vi "device on off list mouse down.vi"(6 "Button":u16, 7 "Coords":T1, 9 "Array 2":i32[](array[numeric]), 10 "CtlRef":refnum<vi>, 11 "Array in":refnum<vi>) -> (2 "Array":bool[](array[boolean]), 3 "ItemSyms":i32[](array[numeric]))   [LabVIEW 2018]
uses:
  <vilib>/Utility/miscctls.llb/LVPoint32TypeDef.ctl
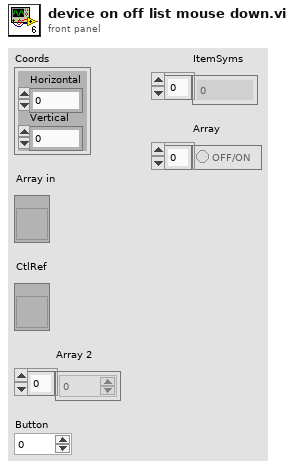
[diagram p1: front panel]
types:
  T1 = typedef "LVPoint32TypeDef.ctl" = cluster{"Horizontal":i32, "Vertical":i32}
  T2 = enum8{"Enabled", "Disabled", "Disabled and Grayed Out"}
  T3 = typedef "mysql_authentication.ctl" = cluster{"User":string, "Password":string, "Database":string}
  T4 = cluster{"Port":u16, "IP Address":string, "Authentication":T3}
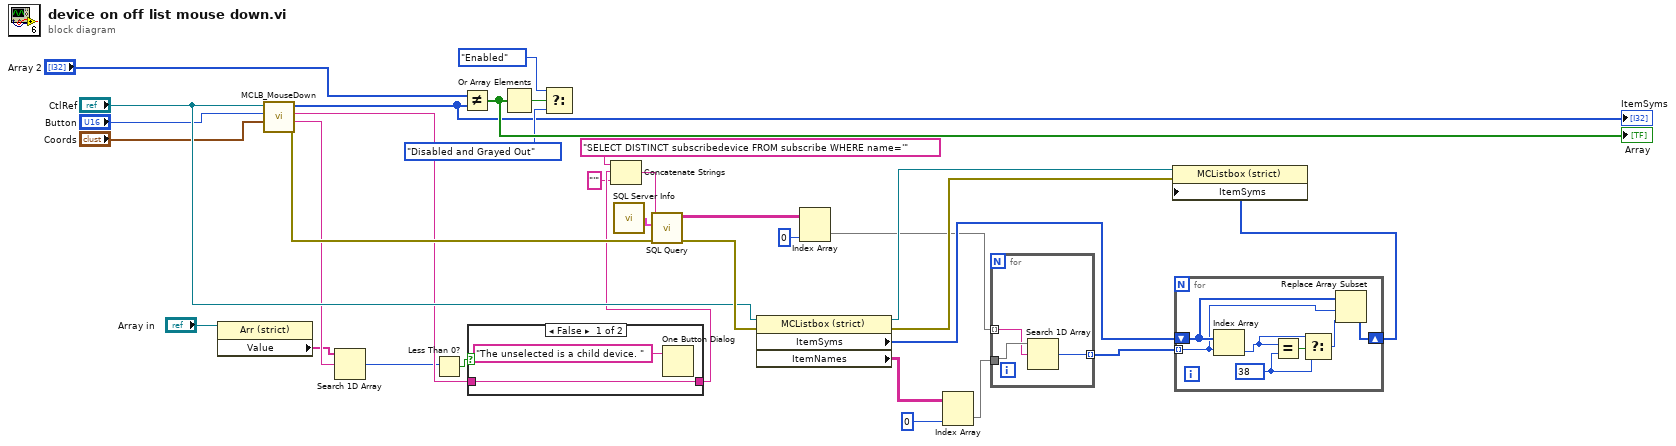
[diagram p0: block diagram]
diagram:
  n1 = property class="Arr (strict)"(reference="Array in") -> ("Value"=w10:string[])  [unwired: 1 in, 2 out]
  n2 = call "MCLB_MouseDown.vi"("Coords"="Coords", "Button"="Button", "MCListbox Refnum"="CtlRef") -> ("error out"=w31:errorcluster, "Unselected Item"=w11:string, "Selected Item"=w13:string, "ItemSyms"=w4:i32[])  [unwired: 5 in]
  "ItemSyms" <- w4
  n3 = Search 1D Array(1D array=w10, element=w11) -> (index of element=w9:i32)  [unwired: 1 in]
  n4 = Less Than 0?(x=w9) -> (x < 0?=w12:bool)
  n5 = Not Equal?(x="Array 2", y=w4) -> (x != y?=w8:bool[])
  "Array" <- w8
  n6 = case shown="False" w12 {
    tunnel: w13 -> [w35 w36]
    tunnel: [w35 w36] -> w20
    frame False {
      n7 = One Button Dialog(message="The unselected is a child device. ") -> ()  [unwired: 1 in, 1 out]
    }
    frame True {
    }
  }
  n8 = Or Array Elements(Boolean array=w8) -> (logical OR=w33:bool)
  n9 = Select(t=T2."Enabled" ("Disabled"), s=w33, f=T2."Disabled and Grayed Out" ("Disabled")) -> ()  [unwired: 1 out]
  n10 = Concatenate Strings("SELECT DISTINCT subscribedevice FROM subscribe WHERE name='" ("Query"), w20, "'" ("string")) -> (w16:string)
  n11 = call "SQL Server Info.vi"() -> ("SQL Server Info"=w19:T4)
  n12 = call "SQL Query.vi"("error in (no error)"=w31, "SQL Server Info"=w19, "Query"=w16) -> ("error out"=w32:errorcluster, "data"=w15:string[][])  [unwired: 7 in]
  n13 = property class="MCListbox (strict)"(reference="CtlRef", error in=w32) -> (reference out=w28:refnum<vi>, error out=w29:errorcluster, "ItemSyms"=w26:i32[], "ItemNames"=w24:string[][])
  n14 = Index Array(array=w15, index (col)=0 ("disabled index (col)")) -> (element=w25:string[])  [unwired: 1 in]
  n15 = Index Array(array=w24, index (col)=0 ("disabled index (col)")) -> (element=w22:string[])  [unwired: 1 in]
  n16 = for {
    tunnel: w25 -> [w38] mode=indexing
    tunnel: w22 -> [w39]
    tunnel: [w37] -> w27 mode=indexing
    n17 = Search 1D Array(1D array=w39, element=w38) -> (index of element=w37:i32)  [unwired: 1 in]
  }
  n18 = for {
    shift-right: [w41] -> w30
    shift-left: w26 -> [w44]
    tunnel: w27 -> [w43] mode=indexing
    w45 = 38
    n19 = Index Array(array=w44, index=w43) -> (element=w40:i32)
    n20 = Equal?(x=w40, y=w45) -> (x = y?=w46:bool)
    n21 = Select(t=w40, s=w46, f=w45) -> (s? t:f=w42:i32)
    n22 = Replace Array Subset(array=w44, new element=w42, index=w43) -> (w41:i32[])
  }
  n23 = property class="MCListbox (strict)"(reference=w28, error in=w29, "ItemSyms"=w30) -> ()  [unwired: 2 out]
